vi "FPGA_SingleApproach.vi"() -> ()   [LabVIEW 2014]
uses:
  <vilib>/Platform/TimedLoop/XDataNode/timing_clust.ctl
  <vilib>/Platform/TimedLoop/XDataNode/nitl_modes.ctl
  <vilib>/Platform/TimedLoop/XDataNode/wakeup.ctl
  <vilib>/rvi/eio/common/nirviEmuTemplateMethod_errors.vi
  <vilib>/rvi/Emulation/niFpgaGetClockAttributes.vi
  <vilib>/rvi/Emulation/niFpgaSctlEmulationGetInTimedLoop.vi
  <vilib>/rvi/Emulation/niFpgaEmulationReportErrorSimple.vi
  <vilib>/rvi/Emulation/niFpgaCriticalErrorInLSC.vi
  <vilib>/eio/EIONode/EIONode.xnode
  <vilib>/Platform/TimedLoop/XDataNode/XDataNode.xnode
  <vilib>/Platform/TimedLoop/XDataNode/XDNodeRunTimeDep.lvlib
panel:
  in  "Sleep us":i32
  in  "ThresMultiplier":i16
  out "Approached?":bool
  out "PIZRangeExceeded?":bool
  out "RealPIZPos":i16
  out "PresCurr":i16
  in  "stop":bool
  out "ZCalPos":i32
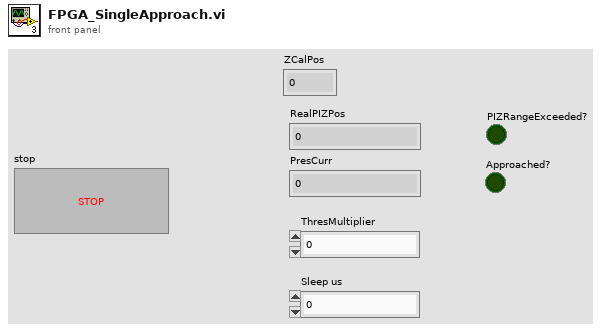
[diagram p1: front panel]
types:
  T1 = typedef "XDNodeRunTimeDep.lvlib/timing_clust.ctl" = cluster{"Expected End [f-1]":u64, "Actual End [f-1]":u64, "Finished Late? [f-1]":bool, "Expected End [i-1]":u64, "Actual End [i-1]":u64, "Finished Late? [i-1]":bool, "Expected Start [i]":u64, "Actual Start [i]":u64, "Expected Start [f]":u64, "Actual Start [f]":u64, "Source Name":string, "Structure Name":string, "Period":i64, "Deadline":i64, "Offset":i64, "Start":i64, "Priority":i32, "Timeout":i32, "Mode":T2, "Wakeup Reason":T3, "Error":errorcluster, "Source Type":string, "Secondary Source Type":string, "Global End Time":u64, "Global Start Time":u64, "Frame Duration":u64, "Iteration Duration":u64, "Assigned CPU":i32, "I/O Scan Engine Mode":u32}
  T2 = typedef "XDNodeRunTimeDep.lvlib/nitl_modes.ctl" = enum32{"No Change", "Process missed periods, maintain original phase", "Discard missed periods, maintain original phase", "Process missed periods, ignore original phase", "Discard missed periods, ignore original phase"}
  T3 = typedef "XDNodeRunTimeDep.lvlib/wakeup.ctl" = enum32{"Normal", "Aborted", "Asynchronous wakeup", "Timing source error", "Timed loop error", "Timeout"}
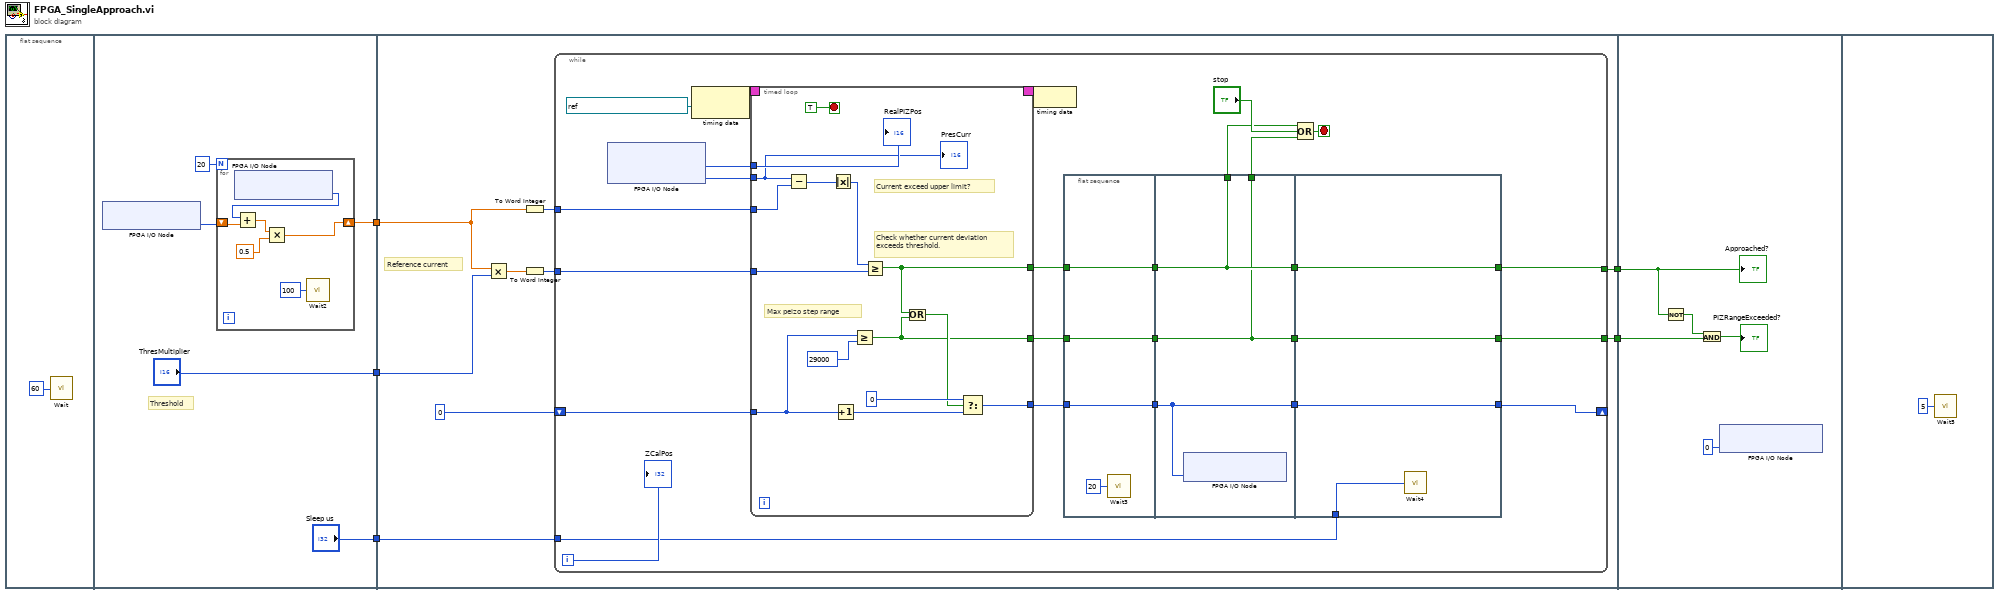
[diagram p0: block diagram]
diagram:
  n1 = flat-sequence {
    tunnel: [w9] -> w5
    tunnel: ["ThresMultiplier"] -> w2
    tunnel: ["Sleep us"] -> w1
    tunnel: [w25] -> w4
    tunnel: [w24] -> w3
    tunnel: w5 -> [w21]
    tunnel: w2 -> [w19]
    tunnel: w1 -> [w18]
    tunnel: w4 -> [w87]
    tunnel: w3 -> [w89]
    frame #0 {
      n2 = call "Wait"("Count(uSec)"=u32 60) -> ()  [unwired: 1 out]
    }
    frame #1 {
      # "Threshold"
      n3 = xnode "FPGA I/O Node"() -> ("Connector0/AI1"=w10:i16)  [unwired: 1 in, 1 out]
      n4 = for {
        N: 20 -> [_]
        shift-right: [w13] -> w9
        shift-left: w10 -> [w17]
        n5 = xnode "FPGA I/O Node"() -> ("Connector0/AI1"=w16:i16)  [unwired: 1 in, 1 out]
        n6 = Add(x=w16, y=w17) -> (x+y=w15:sgl)
        n7 = Multiply(x=w15, y=sgl 0.5) -> (x*y=w13:sgl)
        n8 = call "Wait2"("Count(uSec)"=u32 100) -> ()  [unwired: 1 out]
      }
    }
    frame #2 {
      # "Reference current"
      n9 = Multiply(x=w21, y=w19) -> (x*y=w23:sgl)
      n10 = To Word Integer(number=w21) -> (16bit integer=w20:i16)
      n11 = To Word Integer(number=w23) -> (16bit integer=w22:i16)
      n12 = while {
        tunnel: w22 -> [w44]
        tunnel: w20 -> [w43]
        tunnel: [w32] -> w25
        tunnel: [w31] -> w24
        shift-right: [w29] -> _
        shift-left: i16 0 -> [w45]
        tunnel: w18 -> [w27]
        i -> [w28]
        stop <- w46 stop-if-true
        n13 = xnode "FPGA I/O Node"() -> ("Connector0/AI0"=w49:i16, "Connector0/AI1"=w48:i16)  [unwired: 2 in, 2 out]
        n14 = node-c288(refnum<k21> "40 MHz Onboard Clock" ("Source Name")) -> (w52:T1)
        n15 = timed-loop {
          timing: w52 -> [_]
          timing-out: [_] -> w51
          tunnel: w43 -> [w64]
          tunnel: w44 -> [w66]
          tunnel: w49 -> [w77]
          tunnel: w48 -> [w65]
          tunnel: [w68] -> w37
          tunnel: w45 -> [w70]
          tunnel: [w74] -> w41
          tunnel: [w71] -> w39
          stop <- TRUE stop-if-true
          # "Current exceed upper limit?"
          # "Max peizo step range"
          # "Check whether current deviation\nexceeds threshold."
          n16 = Subtract(x=w65, y=w64) -> (x-y=w67:i16)
          n17 = Absolute Value(x=w67) -> (abs(x)=w69:i16)
          n18 = Increment(x=w70) -> (x+1=w76:i16)
          n19 = Greater Or Equal?(x=w70, y=i16 29000) -> (x >= y?=w71:bool)
          n20 = Greater Or Equal?(x=w69, y=w66) -> (x >= y?=w68:bool)
          n21 = Or(x=w68, y=w71) -> (x .or. y?=w73:bool)
          n22 = Select(t=i16 0, s=w73, f=w76) -> (s? t:f=w74:i16)
          "RealPIZPos" <- w77
          "PresCurr" <- w65
        }
        n23 = node-c288(w51) -> ()
        n24 = flat-sequence {
          tunnel: [w55] -> w42
          tunnel: w41 -> [w55]
          tunnel: [w54] -> w40
          tunnel: w39 -> [w54]
          tunnel: [w53] -> w38
          tunnel: w37 -> [w53]
          tunnel: w42 -> [w57]
          tunnel: w40 -> [w58]
          tunnel: w38 -> [w59]
          tunnel: [w59] -> w36
          tunnel: [w58] -> w35
          tunnel: [w59] -> w34
          tunnel: [w58] -> w33
          tunnel: [w57] -> w30
          tunnel: w34 -> [w63]
          tunnel: w33 -> [w62]
          tunnel: [w63] -> w32
          tunnel: [w62] -> w31
          tunnel: w30 -> [w61]
          tunnel: [w61] -> w29
          tunnel: w27 -> [w60]
          frame #0 {
            n25 = call "Wait3"("Count(uSec)"=u32 20) -> ()  [unwired: 1 out]
          }
          frame #1 {
            n26 = xnode "FPGA I/O Node"("Connector0/AO0"=w57) -> ()  [unwired: 1 in, 1 out]
          }
          frame #2 {
            n27 = call "Wait4"("Count(uSec)"=w60) -> ()  [unwired: 1 out]
          }
        }
        n28 = Compound Arithmetic op=OR(w36, "stop", w35) -> (w46:bool)
        "ZCalPos" <- w28
      }
    }
    frame #3 {
      n29 = Not(x=w87) -> (.not. x?=w86:bool)
      n30 = And(x=w86, y=w89) -> (x .and. y?=→"PIZRangeExceeded?":bool)
      n31 = xnode "FPGA I/O Node"("Connector0/AO0"=i16 0) -> ()  [unwired: 1 in, 1 out]
      "Approached?" <- w87
    }
    frame #4 {
      n32 = call "Wait5"("Count(mSec)"=u32 5) -> ()  [unwired: 1 out]
    }
  }
